vi "ALTS-2015 Bundle Cluster for DB Result format.vi"(7 "Options":T1, 8 "error in (no error)":errorcluster, 11 "Station Enum":T3) -> (0 "error out":errorcluster, 3 "DB Result Cluster Out":T2)   [LabVIEW 2013]
doc: "Copyright © 2005, Soliton Technologies.\nAll rights reserved."
uses:
  Controls/ALTS-2015 Station Cluster.ctl
  Controls/ALTS-2015 DB Result Cluster.ctl
  Controls/ALTS-2015 Bundle Cluster for DB Result Options.ctl
  Controls/ALTS-2015 LV2GBL Station Info Options.ctl
panel:
  in  "DB Result Cluster":T2
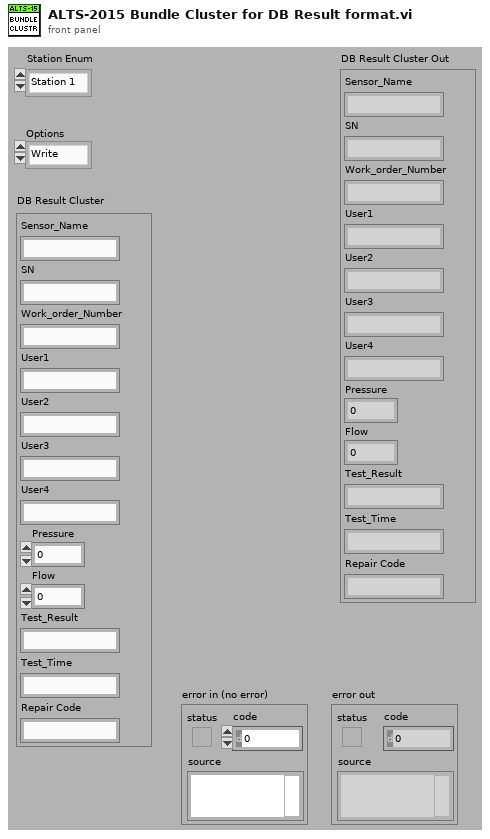
[diagram p1: front panel]
types:
  T1 = typedef "ALTS-2015 Bundle Cluster for DB Result Options.ctl" = enum16{"Write", "Read"}
  T2 = typedef "ALTS-2015 DB Result Cluster.ctl" = cluster{"Sensor_Name":string, "SN":string, "Work_order_Number":string, "User1":string, "User2":string, "User3":string, "User4":string, "Pressure":dbl, "Flow":dbl, "Test_Result":string, "Test_Time":string, "Repair Code":string}
  T3 = typedef "ALTS-2015 Station Cluster.ctl" = enum16{"Station 1", "Station 2", "Station 3", "Station 4"}
  T4 = typedef "ALTS-2015 LV2GBL Station Info Options.ctl" = enum16{"Init", "Read", "Read All", "Write Sensor ID", "Write  WO & SN", "Write Test Data", "Write Station Status", "Write Station Occupancy", "Write Rerun", "Clear All", "Clear Test Result"}
  T5 = typedef "ALTS-2015 Station Details.ctl" = cluster{"Station Number":string, "Work Order Number":string, "Sensor Name":string, "Pressure (PSI)":string, "Flow (SCCM)":string, "Test Time ":string, "Test Result":string, "Serial Number":string, "Station Status":T6, "Station Occupied?":bool, "Rerun Count":i32, "Test Type":i32}
  T6 = typedef "ALTS-2015 Status Ring Indicator.ctl" = u16
  T7 = typedef "ALTS-2015 User Info Cluster.ctl" = cluster{"User 1":string, "User 2":string, "User 3":string, "User 4":string}
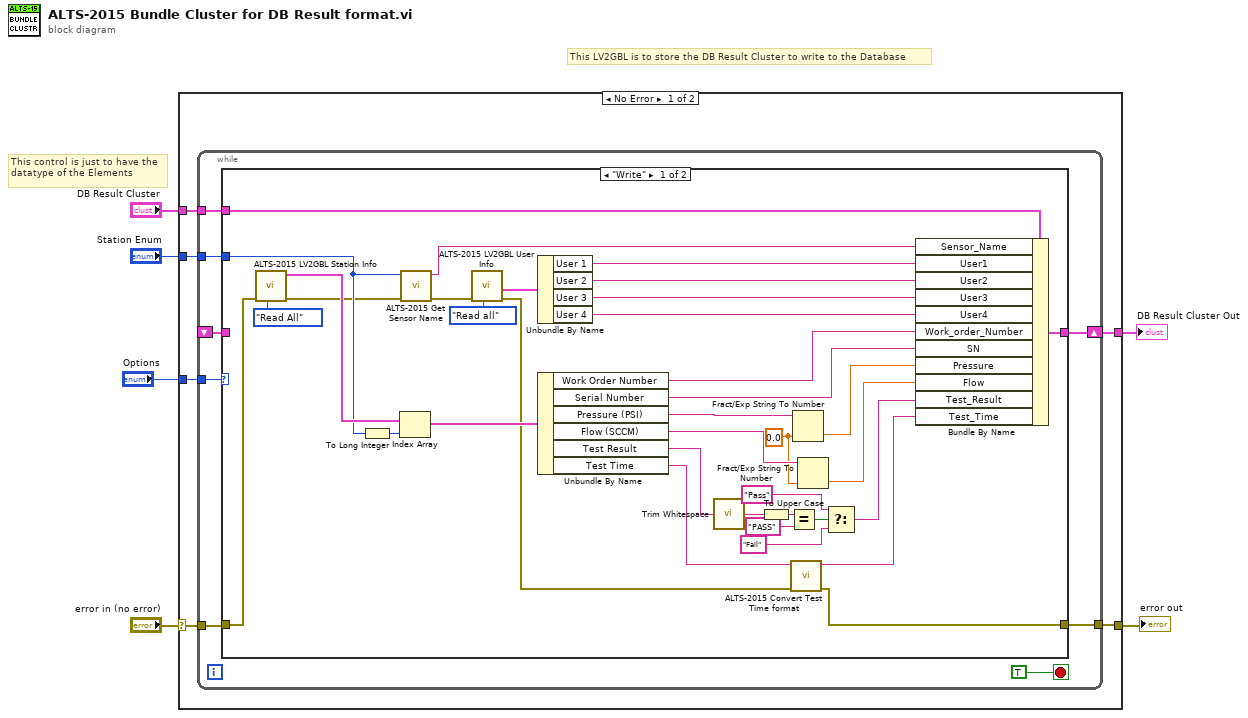
[diagram p0: block diagram]
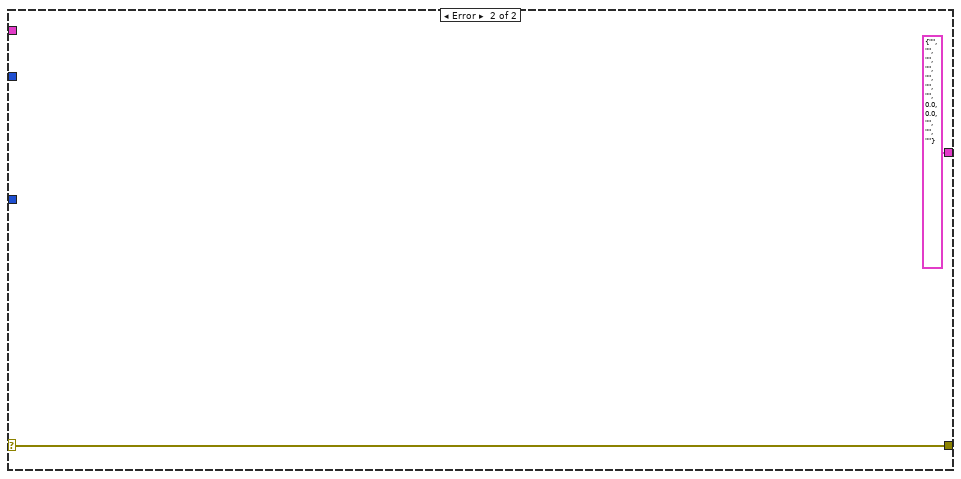
[diagram p3: hidden frame]
diagram:
  # "This LV2GBL is to store the DB Result Cluster to write to the Database"
  # "This control is just to have the datatype of the Elements"
  n1 = case shown="No Error" "error in (no error)" {
    selector: "error in (no error)" -> [w10 w60]
    tunnel: [w9 w60] -> w5
    tunnel: "Station Enum" -> [w12 _]
    tunnel: [w11 T2 {"Sensor_Name"="", "SN"="", "Work_order_Number"="", "User1"="", "User2"="", "User3"="", "User4"="", "Pressure"=0.0, "Flow"=0.0, "Test_Result"="", "Test_Time"="", "Repair Code"=""} ("DB Result Cluster")] -> w3
    tunnel: "Options" -> [w8 _]
    tunnel: "DB Result Cluster" -> [w7 _]
    frame No Error {
      n2 = while {
        tunnel: w12 -> [w20]
        tunnel: w10 -> [w18]
        tunnel: [w17] -> w9
        tunnel: w8 -> [w16]
        shift-right: [w19] -> w11
        shift-left: _ -> [w14]
        tunnel: w7 -> [w13]
        stop <- TRUE stop-if-true
        n3 = case shown="\"Write\"" w16 {
          tunnel: w20 -> [w50 _]
          tunnel: [w37 w58] -> w19
          tunnel: [w25 w57] -> w17
          tunnel: w18 -> [w24 w57]
          tunnel: w14 -> [_ w58]
          tunnel: w13 -> [w34 _]
          frame "Write" {
            w26 = 0.0
            n4 = call "ALTS-2015 LV2GBL Station Info.vi"("Options"=ALTS-2015_LV2GBL_Station_Info_Options."Read All", "error in"=w24) -> ("error out"=w22:errorcluster, "Station Info Array"=w53:T5[])  [unwired: 7 in, 1 out]
            n5 = To Long Integer(number=w50) -> (32bit integer=w52:i32)
            n6 = Index Array(array=w53, index=w52) -> (element=w51:T5)
            n7 = call "ALTS-2015 Get Sensor Name.vi"("error in (no error)"=w22, "Station Enum"=w50) -> ("error out"=w23:errorcluster, "Sensor Name"=w49:string)  [unwired: 8 in]
            n8 = call "ALTS-2015 LV2GBL User Info.vi"("Options"=enum16{"Read all", "Write all"}."Read all", "error in"=w23) -> ("error out"=w21:errorcluster, "User Info Out"=w56:T7)  [unwired: 8 in]
            n9 = Unbundle By Name(w56) -> ("User 1"=w48:string, "User 2"=w47:string, "User 3"=w46:string, "User 4"=w45:string)
            n10 = Unbundle By Name(w51) -> ("Work Order Number"=w36:string, "Serial Number"=w35:string, "Pressure (PSI)"=w41:string, "Flow (SCCM)"=w39:string, "Test Result"=w44:string, "Test Time"=w43:string)
            n11 = call <vilib>:"Trim Whitespace.vi"("string"=w44) -> ("trimmed string"=w33:string)  [unwired: 1 in]
            n12 = To Upper Case(1:w33) -> (0:w32:string)
            n13 = Equal?(x=w32, y="PASS") -> (x = y?=w31:bool)
            n14 = call "ALTS-2015 Convert Test Time format.vi"("error in (no error)"=w21, "String"=w43) -> ("error out"=w25:errorcluster, "Test Time(YYYYMMDDHHMMSS)"=w42:string)  [unwired: 8 in]
            n15 = Fract/Exp String To Number(string=w41, default (0 dbl)=w26) -> (number=w40:dbl)  [unwired: 2 in, 1 out]
            n16 = Fract/Exp String To Number(string=w39, default (0 dbl)=w26) -> (number=w38:dbl)  [unwired: 2 in, 1 out]
            n17 = Select(t="Pass" ("y"), s=w31, f="Fail" ("y")) -> (s? t:f=w29:string)
            n18 = Bundle By Name(cluster=w34, "Sensor_Name"=w49, "User1"=w48, "User2"=w47, "User3"=w46, "User4"=w45, "Work_order_Number"=w36, "SN"=w35, "Pressure"=w40, "Flow"=w38, "Test_Result"=w29, "Test_Time"=w42) -> (w37:T2)
          }
          frame "Read", Default {
          }
        }
      }
    }
    frame Error {
    }
  }
  "error out" <- w5
  "DB Result Cluster Out" <- w3
